vi "closeSharedVariableReferences.vi"(8 "error in (no error)":errorcluster, 11 "Model in":refnum<class "Model.lvclass">) -> (0 "error out":errorcluster, 3 "Model out":refnum<class "Model.lvclass">)   [LabVIEW 2012, in "Model.lvclass"]
doc: "Closes references to the PubDataSVs."
uses:
  Model.lvclass
  Model.lvclass/Model.ctl
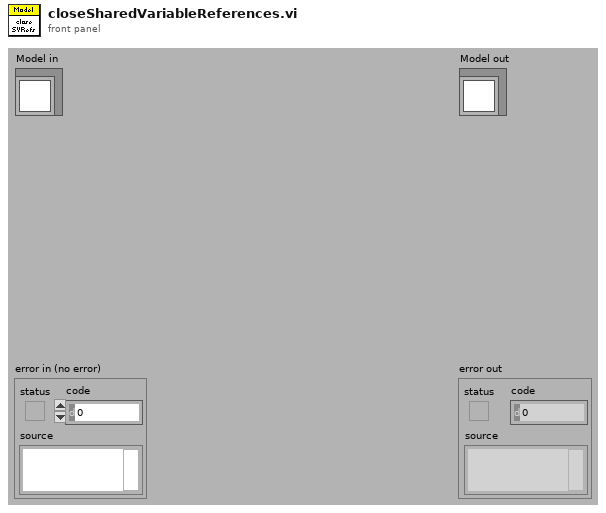
[diagram p1: front panel]
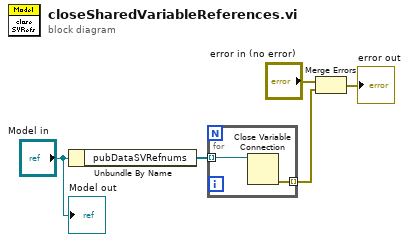
[diagram p0: block diagram]
diagram:
  n1 = Unbundle By Name("Model in") -> ("pubDataSVRefnums"=w5:refnum<k21>[])
  n2 = for {
    tunnel: w5 -> [w7] mode=indexing
    tunnel: [w6] -> w2 mode=indexing
    n3 = Close Variable Connection(11:w7) -> (0:w6:errorcluster)  [unwired: 1 in]
  }
  n4 = Merge Errors("error in (no error)", w2) -> (→"error out":errorcluster)
  "Model out" <- "Model in"
